vi "InitilizeQ.vi"(8 "Error In":errorcluster) -> (0 "Error Out":errorcluster)   [LabVIEW 2017, in "UserInterface.lvlib"]
uses:
  UserInterface.lvlib
  States_FGVQ.ctl
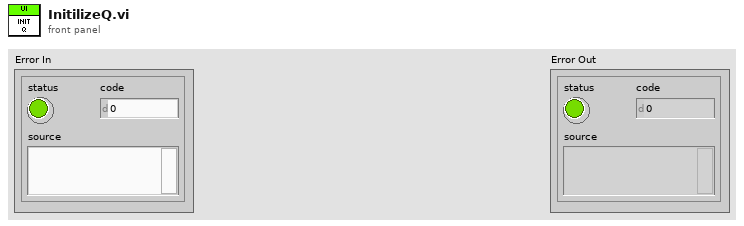
[diagram p1: front panel]
types:
  T1 = typedef "UserInterface.lvlib/States_FGVQ.ctl" = enum16{"Get", "Shutdown", "Initialize"}
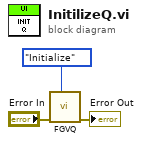
[diagram p0: block diagram]
diagram:
  n1 = call "FGVQ.vi"("State"=States_FGVQ."Initialize", "Error In"="Error In") -> ("Error Out"=→"Error Out":errorcluster)  [unwired: 8 in, 1 out]
